vi "ExportPosList.vi"(8 "error in (no error)":errorcluster, 11 "Array":string[][](array[string])) -> (0 "error out":errorcluster, 3 "XML File Path":path)   [LabVIEW 2018]
uses:
  <vilib>/Utility/xml.llb/Write to XML File(array).vi
  <vilib>/Utility/xml.llb/Read From XML File(array).vi
panel:
  out "XML Elements":string[](array[string])
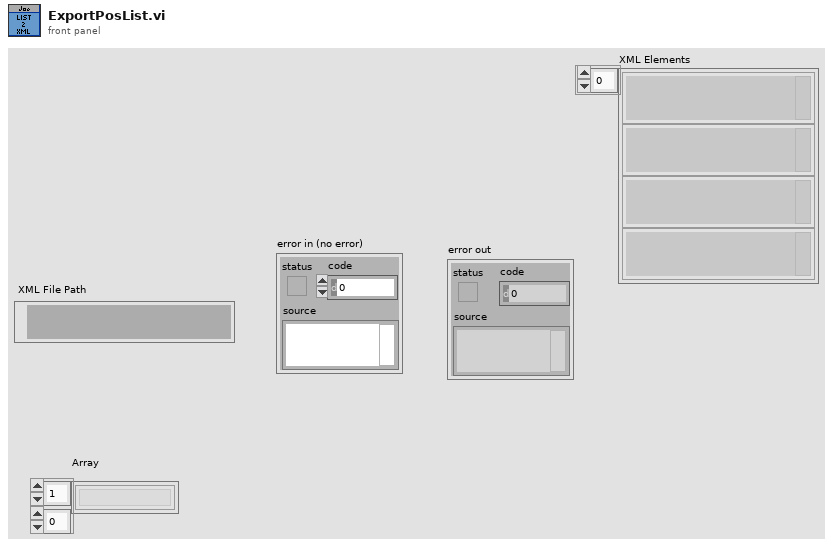
[diagram p1: front panel]
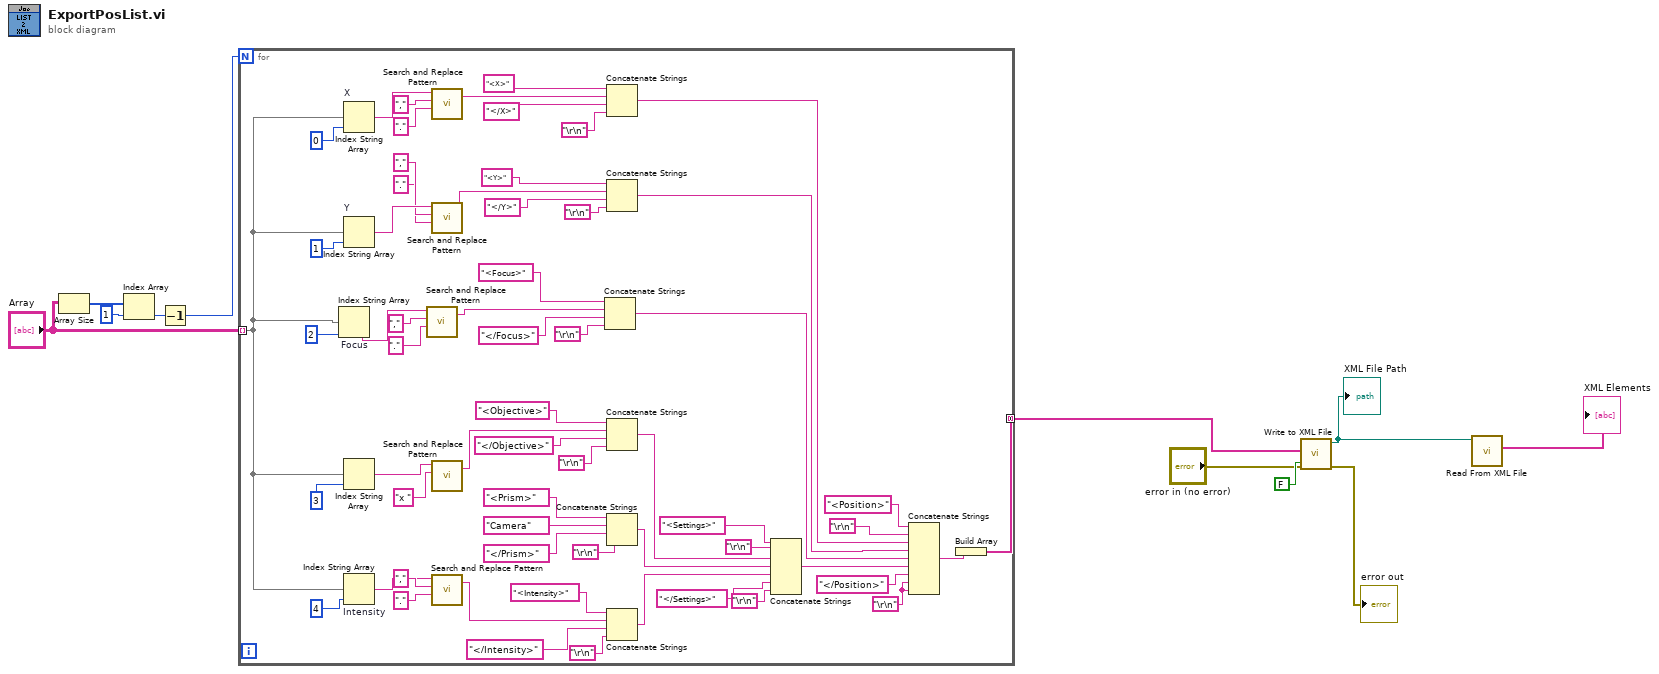
[diagram p0: block diagram]
diagram:
  n1 = Array Size(array="Array") -> (size(s)=w5:i32[])
  n2 = Index Array(array=w5, index=1) -> (element=w3:i32)
  n3 = Decrement(x=w3) -> (x-1=w8:i32)
  n4 = for {
    N: w8 -> [_]
    tunnel: "Array" -> [w13] mode=indexing
    tunnel: [w59] -> w11 mode=concatenating
    w37 = "\r\n"
    n5 = Index String Array "Focus"(1:2 ("index"), 2:w13) -> (0:w20:string)  [unwired: 1 in]
    n6 = Index String Array "X"(1:0 ("index"), 2:w13) -> (0:w27:string)  [unwired: 1 in]
    n7 = Index String Array "Y"(1:1 ("index"), 2:w13) -> (0:w33:string)  [unwired: 1 in]
    n8 = Index String Array(1:3 ("index"), 2:w13) -> (0:w36:string)  [unwired: 1 in]
    n9 = Index String Array "Intensity"(1:4 ("index"), 2:w13) -> (0:w23:string)  [unwired: 1 in]
    n10 = call <vilib>:"Search and Replace Pattern.vi"("string"=w20, "regular expression (\"\")"="," ("regular expression (\"\")"), "replace string (\"\")"="." ("replace string (\"\")")) -> ("result string"=w21:string)  [unwired: 2 in, 1 out]
    n11 = call <vilib>:"Search and Replace Pattern.vi"("string"=w27, "regular expression (\"\")"="," ("regular expression (\"\")"), "replace string (\"\")"="." ("replace string (\"\")")) -> ("result string"=w26:string)  [unwired: 2 in, 1 out]
    n12 = call <vilib>:"Search and Replace Pattern.vi"("string"=w33, "regular expression (\"\")"="," ("regular expression (\"\")"), "replace string (\"\")"="." ("replace string (\"\")")) -> ("result string"=w30:string)  [unwired: 2 in, 1 out]
    n13 = call <vilib>:"Search and Replace Pattern.vi"("string"=w36, "regular expression (\"\")"="x " ("replace string (\"\")")) -> ("result string"=w34:string)  [unwired: 3 in, 1 out]
    n14 = call <vilib>:"Search and Replace Pattern.vi"("string"=w23, "regular expression (\"\")"="," ("regular expression (\"\")"), "replace string (\"\")"="." ("replace string (\"\")")) -> ("result string"=w22:string)  [unwired: 2 in, 1 out]
    n15 = Concatenate Strings("<Focus>" ("string"), w21, "</Focus>" ("string"), "\r\n") -> (w12:string)
    n16 = Concatenate Strings("<X>" ("string"), w26, "</X>" ("string"), "\r\n") -> (w62:string)
    n17 = Concatenate Strings("<Y>" ("string"), w30, "</Y>" ("string"), "\r\n") -> (w61:string)
    n18 = Concatenate Strings("<Objective>" ("string"), w34, "</Objective>" ("string"), "\r\n") -> (w47:string)
    n19 = Concatenate Strings("<Prism>" ("output string"), "Camera" ("output string"), "</Prism>" ("output string"), "\r\n") -> (w42:string)
    n20 = Concatenate Strings("<Intensity>" ("output string"), w22, "</Intensity>", "\r\n") -> (w38:string)
    n21 = Concatenate Strings("<Settings>" ("string"), "\r\n", w47, w42, w38, "</Settings>" ("string"), "\r\n") -> (w63:string)
    n22 = Concatenate Strings("<Position>" ("string"), "\r\n", w62, w61, w12, w63, "</Position>" ("string"), w37, w37) -> (w60:string)
    n23 = Build Array(w60) -> (w59:string[])
  }
  n24 = call-poly <vilib>:"Write to XML File.vi"("Standalone? (T)"=FALSE, "error in (no error)"="error in (no error)", "XML Input"=w11) -> ("error out"=→"error out":errorcluster, "XML File Path"=w2:path)  [unwired: 6 in, 1 out]
  "XML File Path" <- w2
  n25 = call-poly <vilib>:"Read From XML File.vi"("XML File Path"=w2) -> ("XML Elements"=→"XML Elements":string[])  [unwired: 8 in, 2 out]
